vi "sCMOS_acquire_Save_movie.vi"(0 "t0":dbl, 1 "Frames acquired":i32, 4 "N repeat":i32, 5 "error in":errorcluster, 9 "Image IN":T1, 12 "Number of images":i32=10) -> (14 "Stop?":bool, 15 "Frames acquired out":i32, 18 "N repeat out":i32, 19 "error out":errorcluster)   [LabVIEW 2015]
uses:
  <vilib>/vision/Image Controls.llb/IMAQ Image.ctl
  GLOBAL/Global_ABORT.vi
  GLOBAL/Global_CAMERA.vi
panel:
  in  "Handle":u32
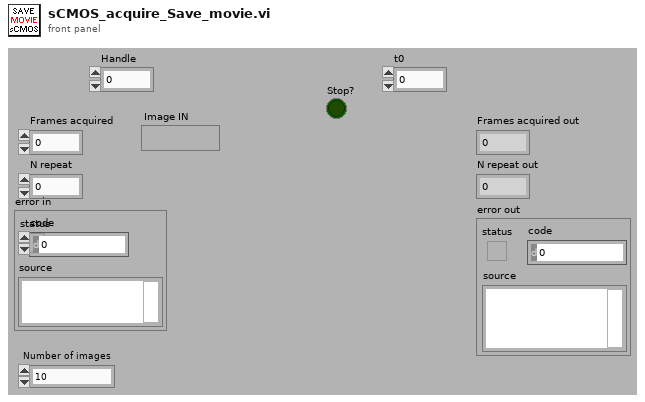
[diagram p1: front panel]
types:
  T1 = typedef "IMAQ Image.ctl" = refnum<image>
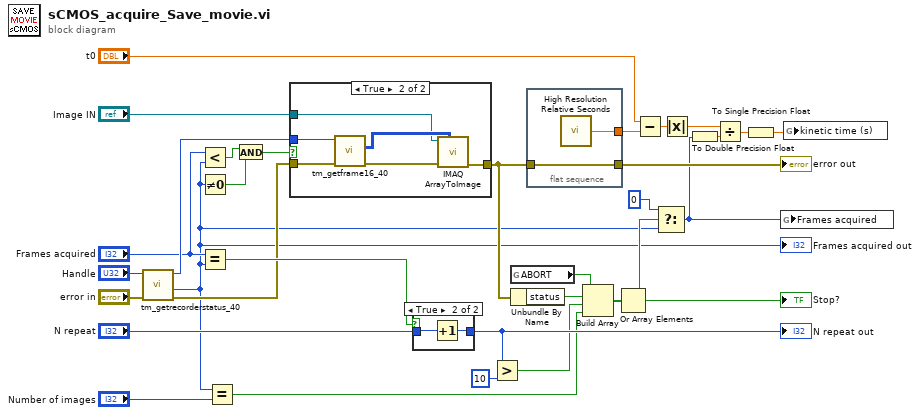
[diagram p0: block diagram]
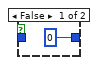
[diagram p3: hidden frame]
diagram:
  n1 = call <userlib>:"tm_getrecorderstatus_40.vi"("error in (no error)"="error in", "Handle"="Handle") -> ("error out"=w18:errorcluster, "Count"=w6:i32, "Handle"=w19:u32)  [unwired: 6 in, 1 out]
  "Frames acquired out" <- w6
  n2 = Less?(x="Frames acquired", y=w6) -> (x < y?=w5:bool)
  n3 = Not Equal To 0?(x=w6) -> (x != 0?=w4:bool)
  n4 = Equal?(x="Frames acquired", y=w6) -> (x = y?=w20:bool)
  n5 = Equal?(x=w6, y="Number of images") -> (x = y?=w26:bool)
  n6 = And(x=w5, y=w4) -> (x .and. y?=w3:bool)
  n7 = case shown="True" w3 {
    tunnel: w19 -> [_ w39]
    tunnel: w18 -> [w33 w38]
    tunnel: "Image IN" -> [_ w35]
    tunnel: [w33 w34] -> w16
    frame False {
    }
    frame True {
      n8 = call <userlib>:"tm_getframe16_40.vi"("error in (no error)"=w38, "Handle in"=w39) -> ("error out"=w36:errorcluster, "Data"=w37:u16[][])  [unwired: 6 in, 2 out]
      n9 = call "IMAQ ArrayToImage"("Image Pixels (U16)"=w37, "error in (no error)"=w36, "Image"=w35) -> ("error out"=w34:errorcluster)  [unwired: 7 in, 1 out]
    }
  }
  n10 = case shown="True" w20 {
    tunnel: "N repeat" -> [_ w42]
    tunnel: [0 w41] -> w30
    frame False {
    }
    frame True {
      n11 = Increment(x=w42) -> (x+1=w41:i32)
    }
  }
  "N repeat out" <- w30
  n12 = Greater?(x=w30, y=10) -> (0:w25:bool)
  n13 = global read "Global_ABORT.vi" "ABORT"() -> (w1:bool)
  n14 = Unbundle By Name(w16) -> ("status"=w24:bool)
  n15 = flat-sequence {
    tunnel: w16 -> [w44]
    tunnel: [w44] -> w15
    tunnel: [w43] -> w14
    frame #0 {
      n16 = call <vilib>:"High Resolution Relative Seconds.vi"() -> ("relative seconds"=w43:dbl)
    }
  }
  n17 = Build Array(w1, w24, w25, w26) -> (w27:bool[])
  n18 = Or Array Elements(Boolean array=w27) -> (logical OR=w23:bool)
  "Stop?" <- w23
  n19 = Subtract(x="t0", y=w14) -> (x-y=w12:dbl)
  n20 = Select(t=0, s=w23, f=w6) -> (s? t:f=w10:i32)
  n21 = Absolute Value(x=w12) -> (abs(x)=w11:dbl)
  n22 = To Double Precision Float(number=w10) -> (double precision float=w8:dbl)
  n23 = Divide(x=w11, y=w8) -> (x/y=w9:dbl)
  n24 = To Single Precision Float(number=w9) -> (single precision float=w2:sgl)
  n25 = global write "Global_CAMERA.vi" "Frames acquired"(w10) -> ()
  n26 = global write "Global_CAMERA.vi" "kinetic time (s)"(w2) -> ()
  "error out" <- w15
